vi "sum of 3 Gaussians with offset.vi"(3 "output control":T1, 4 "data":variant, 5 "X":dbl[](array[numeric]), 6 "a":dbl[](array[numeric])) -> (0 "error out":errorcluster, 1 "f'(X,a)":dbl[][](array[numeric]), 2 "f(X,a)":dbl[](array[numeric]))   [LabVIEW 2011]
uses:
  <vilib>/gmath/NumericalOptimization/LM_output select.ctl
  <vilib>/gmath/NI_Gmath.lvlib
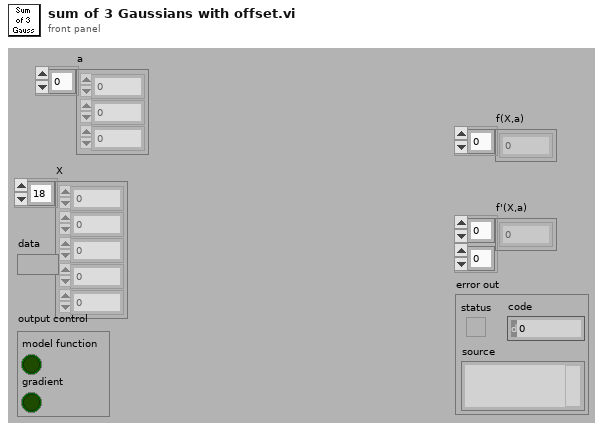
[diagram p1: front panel]
types:
  T1 = typedef "NI_Gmath.lvlib/LM_output select.ctl" = cluster{"model function":bool, "gradient":bool}
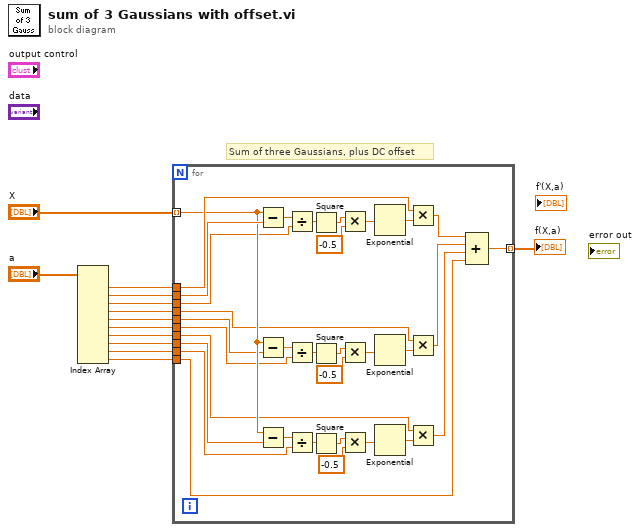
[diagram p0: block diagram]
diagram:
  # "Sum of three Gaussians, plus DC offset"
  n1 = Index Array(array="a") -> (element #1=w12:dbl, element #2=w11:dbl, element #3=w10:dbl, element #4=w9:dbl, element #5=w8:dbl, element #6=w7:dbl, element #7=w6:dbl, element #8=w5:dbl, element #9=w4:dbl, element #10=w3:dbl)  [unwired: 10 in]
  n2 = for {
    tunnel: "X" -> [w38] mode=indexing
    tunnel: w12 -> [w44]
    tunnel: w11 -> [w46]
    tunnel: w10 -> [w24]
    tunnel: w9 -> [w34]
    tunnel: w8 -> [w36]
    tunnel: w7 -> [w23]
    tunnel: w6 -> [w37]
    tunnel: w5 -> [w35]
    tunnel: w4 -> [w22]
    tunnel: w3 -> [w30]
    tunnel: [w29] -> w2 mode=indexing
    n3 = Subtract(x=w38, y=w46) -> (x-y=w25:dbl)
    n4 = Subtract(x=w38, y=w36) -> (x-y=w20:dbl)
    n5 = Subtract(x=w38, y=w35) -> (x-y=w21:dbl)
    n6 = Divide(x=w25, y=w24) -> (x/y=w45:dbl)
    n7 = Divide(x=w20, y=w23) -> (x/y=w41:dbl)
    n8 = Divide(x=w21, y=w22) -> (x/y=w40:dbl)
    n9 = Square(x=w45) -> (x^2=w19:dbl)
    n10 = Square(x=w41) -> (x^2=w18:dbl)
    n11 = Square(x=w40) -> (x^2=w17:dbl)
    n12 = Multiply(x=w19, y=-0.5) -> (x*y=w28:dbl)
    n13 = Multiply(x=w18, y=-0.5) -> (x*y=w27:dbl)
    n14 = Multiply(x=w17, y=-0.5) -> (x*y=w26:dbl)
    n15 = Exponential(1:w28) -> (0:w43:dbl)
    n16 = Exponential(1:w27) -> (0:w42:dbl)
    n17 = Exponential(1:w26) -> (0:w39:dbl)
    n18 = Multiply(x=w44, y=w43) -> (x*y=w33:dbl)
    n19 = Multiply(x=w34, y=w42) -> (x*y=w32:dbl)
    n20 = Multiply(x=w37, y=w39) -> (x*y=w31:dbl)
    n21 = Compound Arithmetic op=ADD(w33, w32, w31, w30) -> (w29:dbl)
  }
  "f(X,a)" <- w2
